vi "RunHighscoreDialog.vi"(8 "error in (no error)":errorcluster, 9 "Engine in":refnum<class "Engine.lvclass">, 10 "GameIn":refnum<class "Game.lvclass">, 11 "Highscore in":refnum<class "Highscore.lvclass">) -> (0 "error out":errorcluster, 1 "Engine out":refnum<class "Engine.lvclass">, 2 "GameOut":refnum<class "Game.lvclass">, 3 "Highscore out":refnum<class "Highscore.lvclass">)   [LabVIEW 2019, in "RT_Game.lvlib" / "Highscore.lvclass"]
uses:
  Highscore.lvclass
  Game/Game.lvclass
  Engine/Engine.lvclass
  Engine/Engine.lvclass/Engine.ctl
  Highscore.lvclass/Highscore.ctl
  HighscoreDialog/HighscoreDialog.lvclass/HighscoreDialog.ctl
  GameObject/GameObject.lvclass/GameObject.ctl
  Menu/States.ctl
  Game/Game.lvclass/Game.ctl
  Game/Write State.vi
  HighscoreDialog/Read IndexInList.vi
  HighscoreDialog/Read CurrName.vi
  GameObject/Read IsActive.vi
  HighscoreDialog/HighscoreDialog.lvclass
  C:/Users/FreshBob/Dropbox/VIs/myRIO_GameConsole/RT/RT_Game/GameObject/GameObject.lvclass
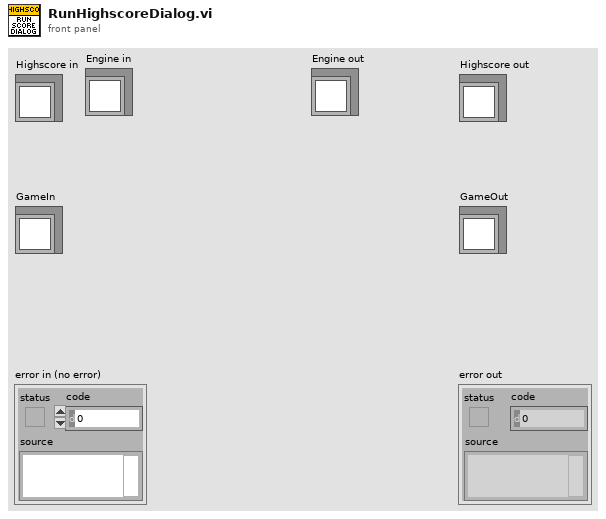
[diagram p1: front panel]
types:
  T1 = typedef "RT_Game.lvlib/Game.lvclass/States.ctl" = enum16{"Init", "Restart", "Menu", "Game", "Resume", "ToggleSingleplayer", "LoadNextGame", "ExitToMenu", "NewHighscore", "GameOver", "SlideOut", "FadeToMenu", "StartFadeToMenu"}
  T2 = typedef "RT_Game.lvlib/Engine.lvclass/Controls.ctl" = cluster{"Controls_1":T3, "Controls_2":cluster{"DirectionX":i8, "DirectionY":i8, "Button1":bool, "Button2":bool}, "SystemButton":bool}
  T3 = typedef "RT_Game.lvlib/Engine.lvclass/ControlPlayer.ctl" = cluster{"DirectionX":i8, "DirectionY":i8, "Button1":bool, "Button2":bool}
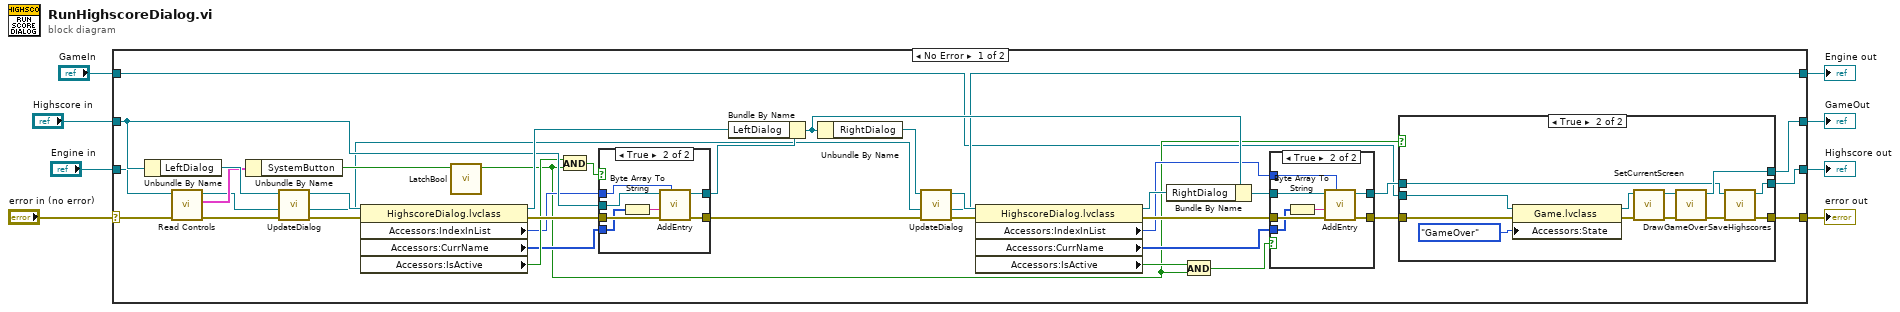
[diagram p0: block diagram]
diagram:
  n1 = case shown="No Error" "error in (no error)" {
    selector: "error in (no error)" -> [w46 w83]
    tunnel: [w20 w83] -> w7
    tunnel: [w16 w82] -> w5
    tunnel: "Highscore in" -> [w32 w82]
    tunnel: "GameIn" -> [w9 w81]
    tunnel: [w19 w81] -> w3
    tunnel: "Engine in" -> [w14 w80]
    tunnel: [w10 w80] -> w1
    frame No Error {
      n2 = Unbundle By Name(w32) -> ("LeftDialog"=w45:refnum<class "HighscoreDialog.lvclass">)
      n3 = call "Read Controls.vi"("error in (no error)"=w46, "Engine in"=w14) -> ("error out"=w15:errorcluster, "Controls"=w13:T2, "Engine out"=w12:refnum<class "Engine.lvclass">)  [unwired: 7 in]
      n4 = Unbundle By Name(w13) -> ("SystemButton"=w29:bool)
      n5 = call "UpdateDialog.vi"("error in (no error)"=w15, "Engine in"=w12, "Highscore in"=w45) -> ("error out"=w43:errorcluster, "Engine out"=w11:refnum<class "Engine.lvclass">, "Highscore out"=w39:refnum<class "HighscoreDialog.lvclass">)  [unwired: 6 in]
      n6 = property class="HighscoreDialog.lvclass"(reference=w39, error in=w43) -> (reference out=w38:refnum<class "HighscoreDialog.lvclass">, error out=w40:errorcluster, "Accessors:IndexInList"=w27:i16, "Accessors:CurrName"=w28:u8[], "Accessors:IsActive"=w31:bool)
      n7 = call "LatchBool.vi"("Boolean"=w29) -> ("Latched Boolean"=w18:bool)  [unwired: 10 in]
      n8 = And(x=w31, y=w18) -> (x .and. y?=w30:bool)
      n9 = case shown="True" w30 {
        tunnel: w40 -> [w71 w79]
        tunnel: [w71 w78] -> w34
        tunnel: [w72 w77] -> w33
        tunnel: w32 -> [w72 w76]
        tunnel: w28 -> [_ w75]
        tunnel: w27 -> [_ w73]
        frame False {
        }
        frame True {
          n10 = Byte Array To String(unsigned byte array=w75) -> (string=w74:string)
          n11 = call "AddEntry.vi"("Index"=w73, "error in (no error)"=w79, "name"=w74, "Highscore in"=w76) -> ("error out"=w78:errorcluster, "Highscore out"=w77:refnum<class "Highscore.lvclass">)  [unwired: 6 in]
        }
      }
      n12 = Bundle By Name(cluster=w33, "LeftDialog"=w38) -> (w41:refnum<class "Highscore.lvclass">)
      n13 = Unbundle By Name(w41) -> ("RightDialog"=w44:refnum<class "HighscoreDialog.lvclass">)
      n14 = call "UpdateDialog.vi"("error in (no error)"=w34, "Engine in"=w11, "Highscore in"=w44) -> ("error out"=w42:errorcluster, "Engine out"=w10:refnum<class "Engine.lvclass">, "Highscore out"=w36:refnum<class "HighscoreDialog.lvclass">)  [unwired: 6 in]
      n15 = property class="HighscoreDialog.lvclass"(reference=w36, error in=w42) -> (reference out=w35:refnum<class "HighscoreDialog.lvclass">, error out=w37:errorcluster, "Accessors:IndexInList"=w23:i16, "Accessors:CurrName"=w24:u8[], "Accessors:IsActive"=w22:bool)
      n16 = Bundle By Name(cluster=w41, "RightDialog"=w35) -> (w25:refnum<class "Highscore.lvclass">)
      n17 = And(x=w22, y=w18) -> (x .and. y?=w21:bool)
      n18 = case shown="True" w21 {
        tunnel: w37 -> [w63 w70]
        tunnel: [w63 w69] -> w26
        tunnel: w25 -> [w62 w68]
        tunnel: [w62 w67] -> w17
        tunnel: w24 -> [_ w66]
        tunnel: w23 -> [_ w64]
        frame False {
        }
        frame True {
          n19 = Byte Array To String(unsigned byte array=w66) -> (string=w65:string)
          n20 = call "AddEntry.vi"("Index"=w64, "error in (no error)"=w70, "name"=w65, "Highscore in"=w68) -> ("error out"=w69:errorcluster, "Highscore out"=w67:refnum<class "Highscore.lvclass">)  [unwired: 6 in]
        }
      }
      n21 = case shown="True" w18 {
        tunnel: w26 -> [w48 w61]
        tunnel: [w48 w52] -> w20
        tunnel: w9 -> [w49 w59]
        tunnel: [w49 w53] -> w19
        tunnel: w17 -> [w47 w51]
        tunnel: [w47 w50] -> w16
        frame False {
        }
        frame True {
          n22 = property class="Game.lvclass"(reference=w59, error in=w61, "Accessors:State"=States."GameOver" ("State")) -> (reference out=w56:refnum<class "Game.lvclass">, error out=w60:errorcluster)
          n23 = call-dynamic "SetCurrentScreen.vi"("error in (no error)"=w60, "Game in"=w56) -> ("error out"=w57:errorcluster, "Game out"=w54:refnum<class "Game.lvclass">)  [unwired: 8 in]
          n24 = call "DrawGameOver.vi"("error in (no error)"=w57, "Game in"=w54) -> ("error out"=w55:errorcluster, "Game out"=w53:refnum<class "Game.lvclass">)  [unwired: 8 in]
          n25 = call "SaveHighscores.vi"("error in (no error)"=w55, "Highscore in"=w51) -> ("error out"=w52:errorcluster, "Highscore out"=w50:refnum<class "Highscore.lvclass">)  [unwired: 8 in]
        }
      }
    }
    frame Error {
    }
  }
  "error out" <- w7
  "Highscore out" <- w5
  "GameOut" <- w3
  "Engine out" <- w1
